vi "CrossCorrelation.vi"   [LabVIEW 2019, in "xy_utilities.lvlib"]
doc: "Compute the cross correlation <b>R_ab</b> of <b>XY-data a</b> and <b>XY-data b</b>.\n\nWire data to the data input to determine the polymorphic instance to use or manually select the instance."
uses:
  xy_utilities.lvlib
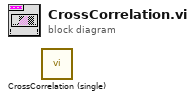
[diagram p0: block diagram]
diagram:
  n1 = call "CrossCorrelation (single).vi"() -> ()  [unwired: 9 in, 3 out]
